vi "Set rate.vi"(7 "[x]":T1, 8 "error in (no error)":errorcluster, 10 "Rate (array)":dbl[](array[numeric]), 11 "Serial Port in":refnum<visa-resource-name>) -> (0 "error out":errorcluster, 3 "Serial Port out":refnum<visa-resource-name>)   [LabVIEW 2016, in "Chemyx_Syringe_Pump_driver.lvlib"]
doc: "Sets the rates of the syringe operations.\n\nRate is an array of double float. Units are those defined by the Set units operation."
uses:
  Chemyx_Syringe_Pump_driver.lvlib
  _private/Control/Control Mode.ctl
panel:
  # "Sets the rates of the syringe"
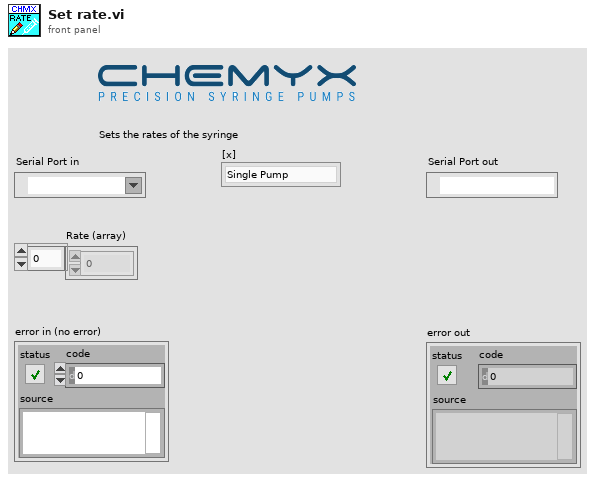
[diagram p1: front panel]
types:
  T1 = typedef "Chemyx_Syringe_Pump_driver.lvlib/Control Mode.ctl" = enum16{"Single Pump", "Pump Chanel 1", "Pump Channel 2", "Cycle Mode"}
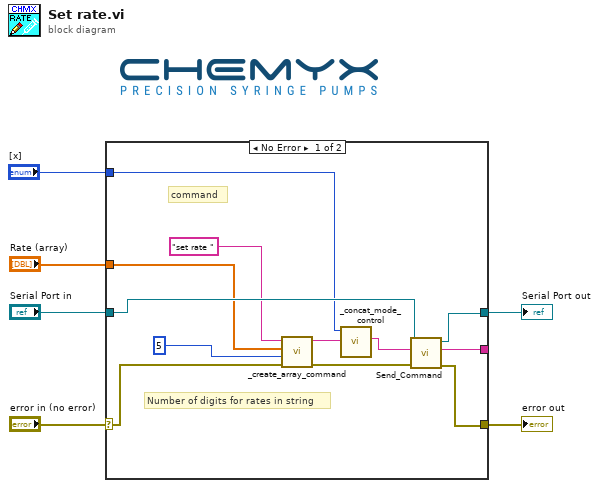
[diagram p0: block diagram]
diagram:
  n1 = case shown="No Error" "error in (no error)" {
    selector: "error in (no error)" -> [w11 w20]
    tunnel: "Serial Port in" -> [w18 w19]
    tunnel: [w17 w20] -> w4
    tunnel: [w16 w19] -> w3
    tunnel: "Rate (array)" -> [w14 _]
    tunnel: [w10 _] -> _
    tunnel: "[x]" -> [w7 _]
    frame No Error {
      # "Number of digits for rates in string"
      # "command"
      n2 = call "_create_array_command.vi"("error in"=w11, "precision (1)"=i16 5 ("precision (6)"), "array"=w14, "Command in"="set rate ") -> ("error out"=w12:errorcluster, "Command out"=w8:string)  [unwired: 6 in]
      n3 = call "_concat_mode_control.vi"("write buffer"=w8, "[x]"=w7) -> ("write buffer out"=w9:string)  [unwired: 9 in]
      n4 = call "Send_Command.vi"("error in (no error)"=w12, "write buffer"=w9, "Serial Port in"=w18) -> ("error out"=w17:errorcluster, "Read buffer"=w10:string, "VISA Refnum out"=w16:refnum<visa-resource-name>)  [unwired: 6 in]
    }
    frame Error {
    }
  }
  "error out" <- w4
  "Serial Port out" <- w3
